vi "Prepare Bus Monitor Interface.vi"(9 "Datum Name":string, 11 "ListboxBusMonitor":refnum<class "ListboxBusMonitor.lvclass">) -> (2 "Valid Transport":refnum<class "ITransport.lvclass">, 3 "SubscriptionPolicy":refnum<class "ISubscriptionPolicy.lvclass">)   [LabVIEW 2018, in "MVA Framework.lvlib" / "ListboxBusMonitor.lvlib" / "ListboxBusMonitor.lvclass"]
doc: "准备总线监视器接口"
uses:
  ListboxBusMonitor.lvclass
  modules/mva-core/Source/SubscriptionPolicy/BasicSubscription/BasicSubscription.lvclass
  modules/composed-transport/Source/Concrete/ActorMessageTransport/ActorMessageTransport.lvclass
  ListboxBusMonitorPanel Messages/Update Monitored Datum Msg/Update Monitored Datum Msg.lvclass
  modules/mva-core/Source/IMediator/ISubscriptionPolicy/ISubscriptionPolicy.lvclass
  modules/composed-transport/Source/ITransport/ITransport.lvclass
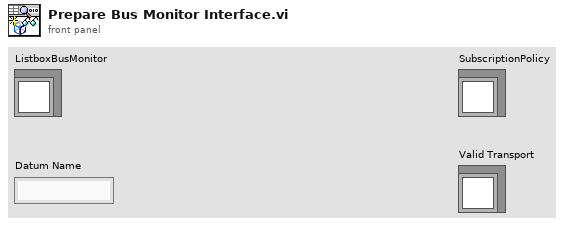
[diagram p1: front panel]
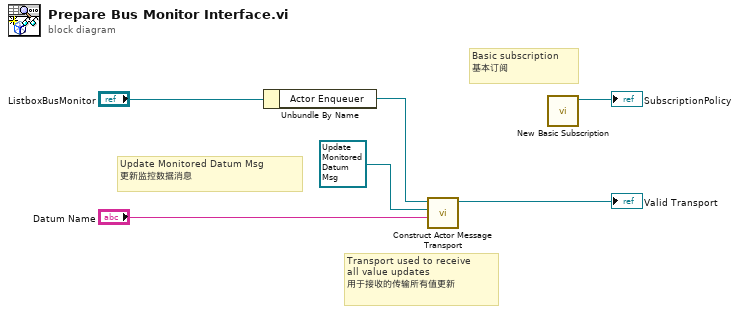
[diagram p0: block diagram]
diagram:
  # "Basic subscription\n基本订阅"
  # "Transport used to receive\nall value updates\n用于接收的传输所有值更新"
  # "Update Monitored Datum Msg\n更新监控数据消息"
  n1 = Unbundle By Name("ListboxBusMonitor") -> ("Actor Enqueuer"=w1:refnum<class "Message Enqueuer.lvclass">)
  n2 = call "Construct Actor Message Transport.vi"("Datum Name"="Datum Name", "Notification Msg"=refnum<class "Update Monitored Datum Msg.lvclass"> refnum ("ListboxBusMonitor.lvlib:Update Monitored Datum Msg.lvclass"), "Message Enqueuer in"=w1) -> ("ActorMessageTransport"=→"Valid Transport":refnum<class "ActorMessageTransport.lvclass">)  [unwired: 7 in, 1 out]
  n3 = call "New Basic Subscription.vi"() -> ("BasicSubscription Out"=→"SubscriptionPolicy":refnum<class "BasicSubscription.lvclass">)  [unwired: 11 in]
